vi "GetTagValue_U32.vi"(6 "error in (no error)":errorcluster caption="Fehler (Eingang, kein Fehler)", 7 "Tag Code":u16, 8 "Directory Entries":T2[](array[typedef]) {"Value" format="%.0x"}, 9 "TIFF file":T1 {"BigTiff,Endian" items=["Big-Endian"=0, "Native"=1, "Little-Endian"=2, "BigTiff-Big-Endian"=256, "Bigtiff,Native"=257, "Biftiff,Littleendian"=258]}) -> (0 "error out":errorcluster caption="Fehler (Ausgang)", 1 "Index (not found = -1)":i32, 2 "Single Value":u32, 3 "TIFF file out":T1 {"BigTiff,Endian" items=["Big-Endian"=0, "Native"=1, "Little-Endian"=2, "BigTiff-Big-Endian"=256, "Bigtiff,Native"=257, "Biftiff,Littleendian"=258]})   [LabVIEW 2011]
uses:
  IFD.ctl
panel:
  out "Valid direct Bytes":u8
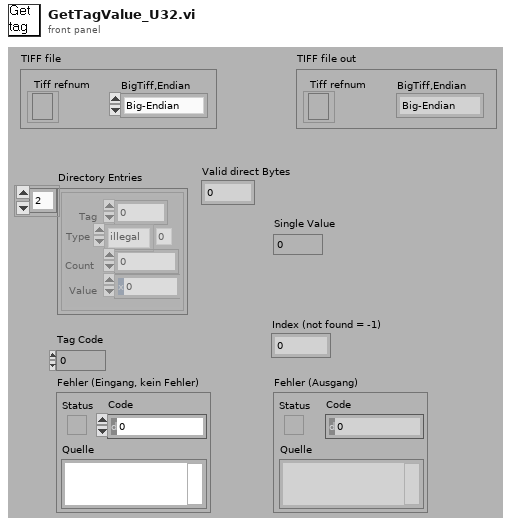
[diagram p1: front panel]
types:
  T1 = cluster{"Tiff refnum":refnum<file>, "BigTiff,Endian":u16}
  T2 = typedef "IFD.ctl" = cluster{"Tag":u16, "Type":enum16{"illegal", "Byte", "Ascii", "Short", "Long", "Rational", "SByte", "Undefined", "SShort", "SLong", "SRational 2xSLong", "Float 4byte", "Double 8Byte", "No13", "No14", "No15", "U64", "I64", "U64-IFD8"}, "Count":u64, "Value":u64}
  T3 = enum16{"illegal", "Byte", "Ascii", "Short", "Long", "Rational", "SByte", "Undefined", "SShort", "SLong", "SRational 2xSLong", "Float 4byte", "Double 8Byte"}[]
  T4 = enum16{"illegal", "Byte", "Ascii", "Short", "Long", "Rational", "SByte", "Undefined", "SShort", "SLong", "SRational 2xSLong", "Float 4byte", "Double 8Byte", "No13", "No14", "No15", "U64", "I64", "U64-IFD8"}
  T5 = cluster{"byte stream type":u32, "byte stream type 2":u32}
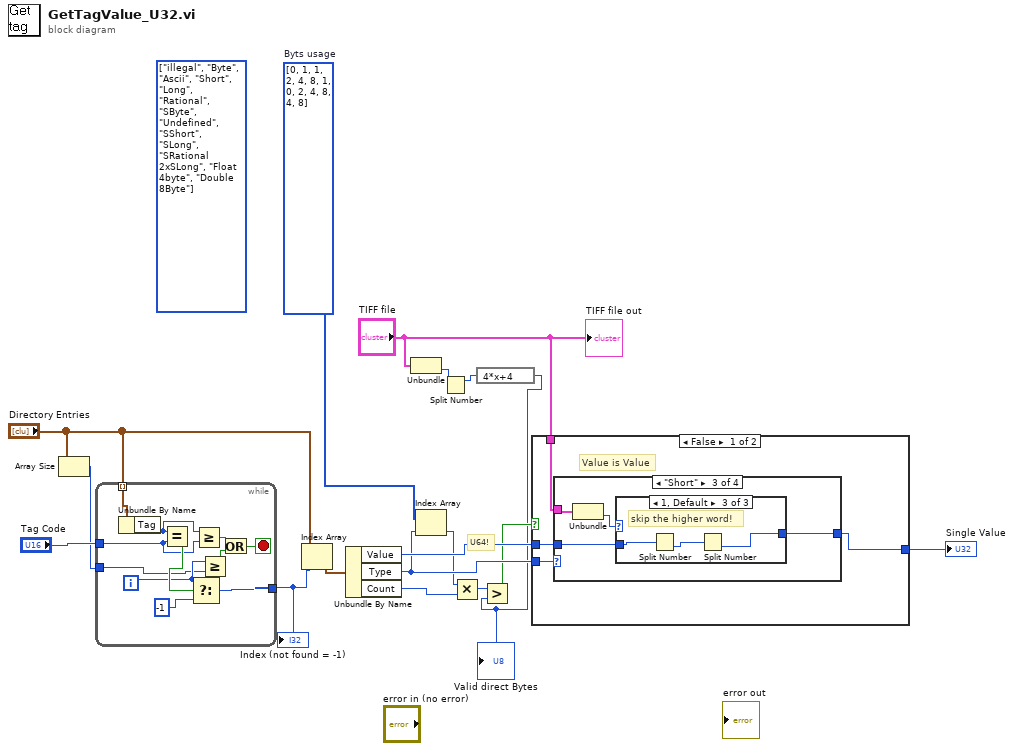
[diagram p0: block diagram]
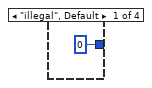
[diagram p2: hidden frame]
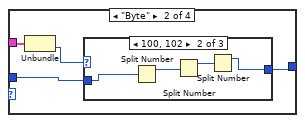
[diagram p3: hidden frame]
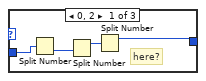
[diagram p4: hidden frame]
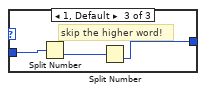
[diagram p5: hidden frame]
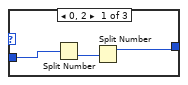
[diagram p6: hidden frame]
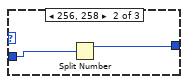
[diagram p7: hidden frame]
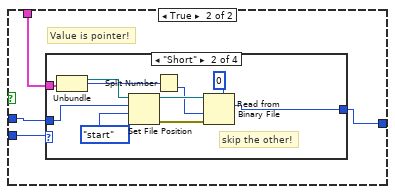
[diagram p9: hidden frame]
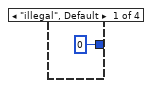
[diagram p10: hidden frame]
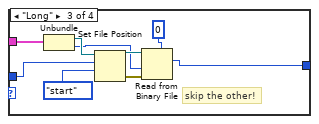
[diagram p11: hidden frame]
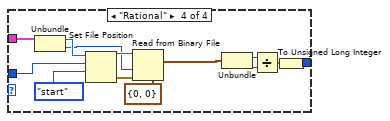
[diagram p12: hidden frame]
diagram:
  w10 = i32[] [0, 1, 1, 2, 4, 8, 1, 0, 2, 4, 8, 4, 8]  # Byts usage
  (unwired) T3 [enum."illegal", enum."Byte", enum."Ascii", enum."Short", enum."Long", enum."Rational", enum."SByte", enum."Undefined", enum."SShort", enum."SLong", enum."SRational 2xSLong", enum."Float 4byte", enum."Double 8Byte"] items=["illegal", "Byte", "Ascii", "Short", "Long", "Rational", "SByte", "Undefined", "SShort", "SLong", "SRational 2xSLong", "Float 4byte", "Double 8Byte"]
  # "U64!"
  n1 = Array Size(array="Directory Entries") -> (size(s)=w12:i32)
  n2 = while {
    tunnel: "Directory Entries" -> [w28] mode=indexing
    tunnel: "Tag Code" -> [w25]
    tunnel: [w23] -> w14
    tunnel: w12 -> [w21]
    i -> [w22]
    stop <- w20 stop-if-true
    n3 = Unbundle By Name(w28) -> ("Tag"=w26:u16)
    n4 = Equal?(x=w26, y=w25) -> (x = y?=w27:bool)
    n5 = Select(t=w22, s=w27, f=-1) -> (s? t:f=w23:i32)
    n6 = Greater Or Equal?(x=w26, y=w25) -> (x >= y?=w19:bool)
    n7 = Greater Or Equal?(x=w22, y=w21) -> (x >= y?=w18:bool)
    n8 = Or(x=w19, y=w18) -> (x .or. y?=w20:bool)
  }
  "Index (not found = -1)" <- w14
  n9 = Index Array(array="Directory Entries", index=w14) -> (element=w16:T2)
  n10 = Unbundle By Name(w16) -> ("Value"=w15:u64, "Type"=w11:T4, "Count"=w8:u64)
  n11 = Unbundle("TIFF file") -> ("BigTiff,Endian"=w3:u16)  [unwired: 1 out]
  n12 = Index Array(array=w10, index=w11) -> (element=w9:i32)
  n13 = Split Number(x=w3) -> (hi(x)=w2:u8)  [unwired: 1 out]
  n14 = Multiply(x=w9, y=w8) -> (x*y=w7:u64)
  n15 = expression code="4*x+4"(w2) -> (w1:u8)
  "Valid direct Bytes" <- w1
  n16 = Greater?(x=w7, y=w1) -> (0:w5:bool)
  n17 = case shown="False" w5 {
    tunnel: w15 -> [w32 w64]
    tunnel: "TIFF file" -> [w31 w65]
    tunnel: w11 -> [w30 w63]
    tunnel: [w29 w62] -> w6
    frame False {
      # "Value is Value"
      n18 = case shown="\"Short\"" w30 {
        tunnel: w31 -> [_ w37 w50 _]
        tunnel: w32 -> [_ w35 w52 w61]
        tunnel: [u32 0 ("Value") w34 w51 w61] -> w29
        frame "illegal", Default {
        }
        frame "Byte" {
          n19 = Unbundle(w37) -> ("BigTiff,Endian"=w36:u16)  [unwired: 1 out]
          n20 = case shown="100, 102" w36 {
            tunnel: w35 -> [w39 w44 w48]
            tunnel: [w40 w42 w46] -> w34
            frame 0, 2 {
              # "here?"
              n21 = Split Number(x=w39) -> (lo(x)=w38:u32)  [unwired: 1 out]
              n22 = Split Number(x=w38) -> (hi(x)=w41:u16)  [unwired: 1 out]
              n23 = Split Number(x=w41) -> (hi(x)=w40:u8)  [unwired: 1 out]
            }
            frame 256, 258 {
              n24 = Split Number(x=w44) -> (hi(x)=w45:u32)  [unwired: 1 out]
              n25 = Split Number(x=w45) -> (hi(x)=w43:u16)  [unwired: 1 out]
              n26 = Split Number(x=w43) -> (hi(x)=w42:u8)  [unwired: 1 out]
            }
            frame 1, Default {
              # "skip the higher word!"
              n27 = Split Number(x=w48) -> (lo(x)=w47:u32)  [unwired: 1 out]
              n28 = Split Number(x=w47) -> (lo(x)=w46:u16)  [unwired: 1 out]
            }
          }
        }
        frame "Short" {
          n29 = Unbundle(w50) -> ("BigTiff,Endian"=w49:u16)  [unwired: 1 out]
          n30 = case shown="1, Default" w49 {
            tunnel: w52 -> [w54 w57 w59]
            tunnel: [w55 w56 w60] -> w51
            frame 0, 2 {
              n31 = Split Number(x=w54) -> (lo(x)=w53:u32)  [unwired: 1 out]
              n32 = Split Number(x=w53) -> (hi(x)=w55:u16)  [unwired: 1 out]
            }
            frame 256, 258 {
              n33 = Split Number(x=w57) -> (hi(x)=w56:u32)  [unwired: 1 out]
            }
            frame 1, Default {
              # "skip the higher word!"
              n34 = Split Number(x=w59) -> (lo(x)=w58:u32)  [unwired: 1 out]
              n35 = Split Number(x=w58) -> (lo(x)=w60:u16)  [unwired: 1 out]
            }
          }
        }
        frame "Long" {
        }
      }
    }
    frame True {
      # "Value is pointer!"
      n36 = case shown="\"Short\"" w63 {
        tunnel: w65 -> [_ w70 w80 w98]
        tunnel: w64 -> [_ w69 w79 w96]
        tunnel: [u32 0 ("Value") w68 w77 w86] -> w62
        frame "illegal", Default {
        }
        frame "Short" {
          # "skip the other!"
          n37 = Unbundle(w70) -> ("Tiff refnum"=w73:refnum<file>, "BigTiff,Endian"=w72:u16)
          n38 = Set File Position(offset (in bytes) (0)=w69, refnum=w73, from (0:start)=enum16{"start", "end", "current"}."start" ("pos mode (0:2)")) -> (refnum out=w75:refnum<file>, error out=w74:errorcluster)  [unwired: 1 in]
          n39 = Split Number(x=w72) -> (lo(x)=w67:u8)  [unwired: 1 out]
          n40 = Read from Binary File(5:u32 0 ("byte stream type"), 8:w74, 9:w67, 11:w75) -> (2:w68:u32)  [unwired: 5 out]
        }
        frame "Long" {
          # "skip the other!"
          n41 = Unbundle(w80) -> ("Tiff refnum"=w82:refnum<file>, "BigTiff,Endian"=w81:u16)
          n42 = Set File Position(offset (in bytes) (0)=w79, refnum=w82, from (0:start)=enum16{"start", "end", "current"}."start" ("pos mode (0:2)")) -> (refnum out=w84:refnum<file>, error out=w83:errorcluster)  [unwired: 1 in]
          n43 = Read from Binary File(5:u32 0 ("byte stream type"), 8:w83, 9:w81, 11:w84) -> (2:w77:u32)  [unwired: 5 out]
        }
        frame "Rational" {
          n44 = Unbundle(w98) -> ("Tiff refnum"=w88:refnum<file>, "BigTiff,Endian"=w87:u16)
          n45 = Set File Position(offset (in bytes) (0)=w96, refnum=w88, from (0:start)=enum16{"start", "end", "current"}."start" ("pos mode (0:2)")) -> (refnum out=w91:refnum<file>, error out=w90:errorcluster)  [unwired: 1 in]
          n46 = Read from Binary File(5:T5 {"byte stream type"=0, "byte stream type 2"=0}, 8:w90, 9:w87, 11:w91) -> (2:w89:T5)  [unwired: 5 out]
          n47 = Unbundle(w89) -> ("byte stream type"=w94:u32, "byte stream type 2"=w93:u32)
          n48 = Divide(x=w94, y=w93) -> (x/y=w92:dbl)
          n49 = To Unsigned Long Integer(number=w92) -> (unsigned 32bit integer=w86:u32)
        }
      }
    }
  }
  "Single Value" <- w6
  "TIFF file out" <- "TIFF file"
